vi "Enviar_configEstacion_Arduino.vi"(0 "VISA resource name":refnum<visa-resource-name>, 5 "Configuracion Estación":T1={"Coordenadas_estacion"={"Coord.Bandeja entrada"={"Coord. X0 entrada"=0, "Coord. Y0 entrada "=0, "Altura Z entrada"=0}, "Coord.Bandeja OK"={"Coord. X0 OK"=0, "Coord. Y0 OK"=0, "Altura Z OK"=0}, "Coord.Bandeja entrada FAIL"={"Coord. X0 FAIL"=0, "Coord. Y0 FAIL"=0, "Altura Z FAIL"=0}, "Coord. Socket"={"Coord. X socket"=0, "Coord. Y socket"=0, "Altura Z socket"=0}}, "Nombre Bandeja"="", "Datos bandeja"={"Nº de columnas "=0, "Nº de filas "=0, "largo"=0, "ancho"=0, "nombre"="nombre", "Paso X (en mm)"=0.0, "Paso Y (en mm)"=0.0, "DISTANCIA SUELO A CHIP  "=0.0, "Nº de celdas totales"=0, "Distancia chips bandejas contiguas"=0.0}}, 11 "error in (no error)":errorcluster) -> (4 "trama datos enviada":string, 6 "datos enviados = datos leídos?":bool, 10 "datos leídos":string, 15 "error IO":errorcluster)   [LabVIEW 2019]
uses:
  LVPROJ_CONFIG_ESTACION/Type_defs/Coordenadas_estacion.ctl
  LVPROJ_CREAR BANDEJAS/Type_defs/Data_Bandeja.ctl
  <vilib>/Utility/error.llb/Error Cluster From Error Code.vi
  <vilib>/ErrorRing/Error Ring.xnode
  SHARED VI'S/SHARED VI'S.lvlib
panel:
  out "return count":u32
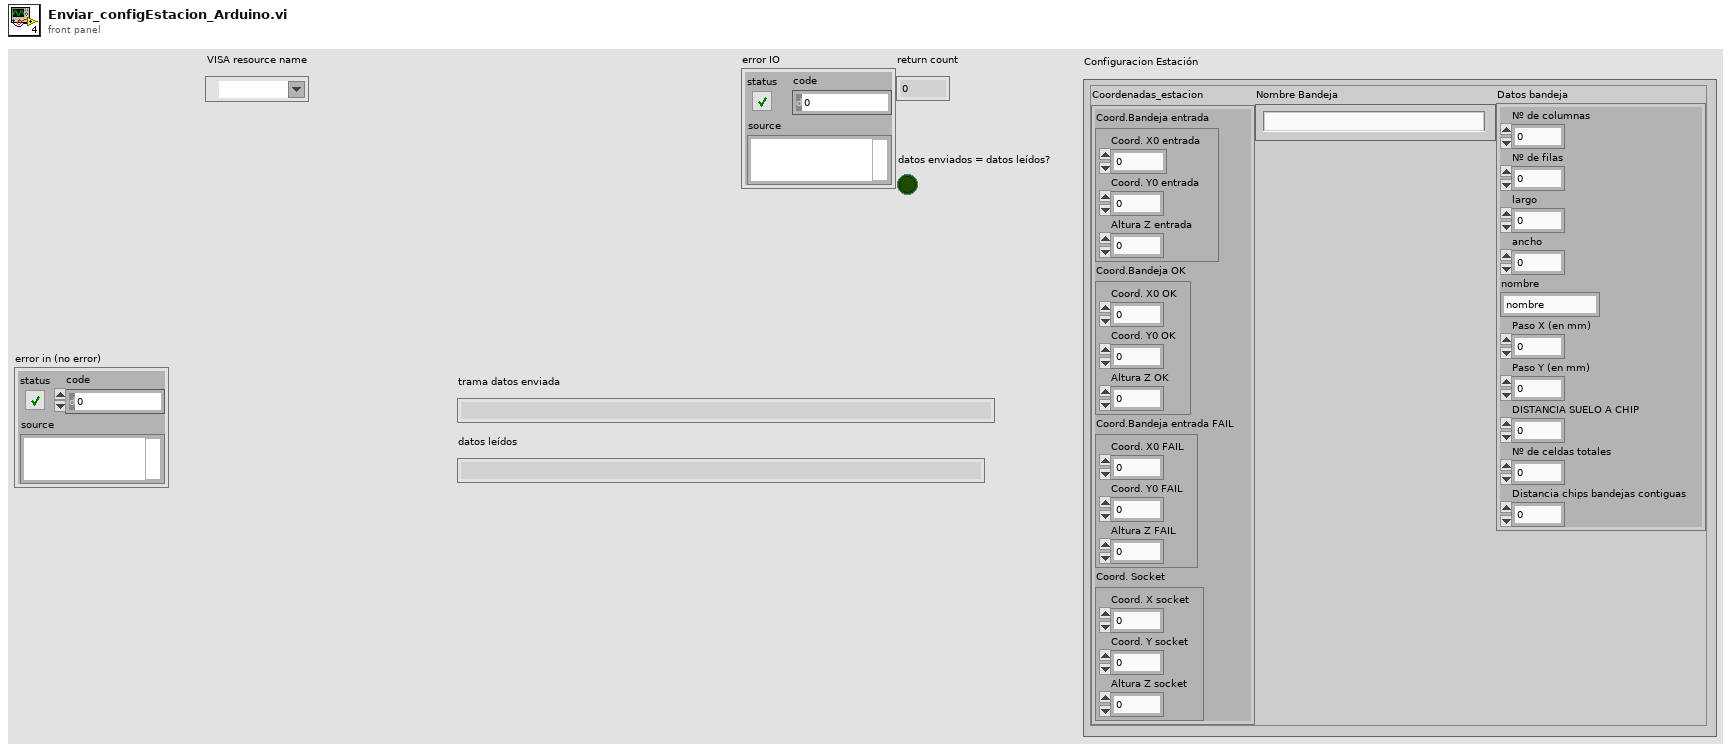
[diagram p1: front panel]
types:
  T1 = typedef "Configuracion_estación.ctl" = cluster{"Coordenadas_estacion":T2, "Nombre Bandeja":string, "Datos bandeja":T3}
  T2 = typedef "Coordenadas_estacion.ctl" = cluster{"Coord.Bandeja entrada":cluster{"Coord. X0 entrada":u32, "Coord. Y0 entrada ":u32, "Altura Z entrada":u32}, "Coord.Bandeja OK":cluster{"Coord. X0 OK":u32, "Coord. Y0 OK":u32, "Altura Z OK":u32}, "Coord.Bandeja entrada FAIL":cluster{"Coord. X0 FAIL":u32, "Coord. Y0 FAIL":u32, "Altura Z FAIL":u32}, "Coord. Socket":cluster{"Coord. X socket":u32, "Coord. Y socket":u32, "Altura Z socket":u32}}
  T3 = typedef "Data_Bandeja.ctl" = cluster{"Nº de columnas ":u32, "Nº de filas ":u32, "largo":u32, "ancho":u32, "nombre":string, "Paso X (en mm)":dbl, "Paso Y (en mm)":dbl, "DISTANCIA SUELO A CHIP  ":dbl, "Nº de celdas totales":u16, "Distancia chips bandejas contiguas":dbl}
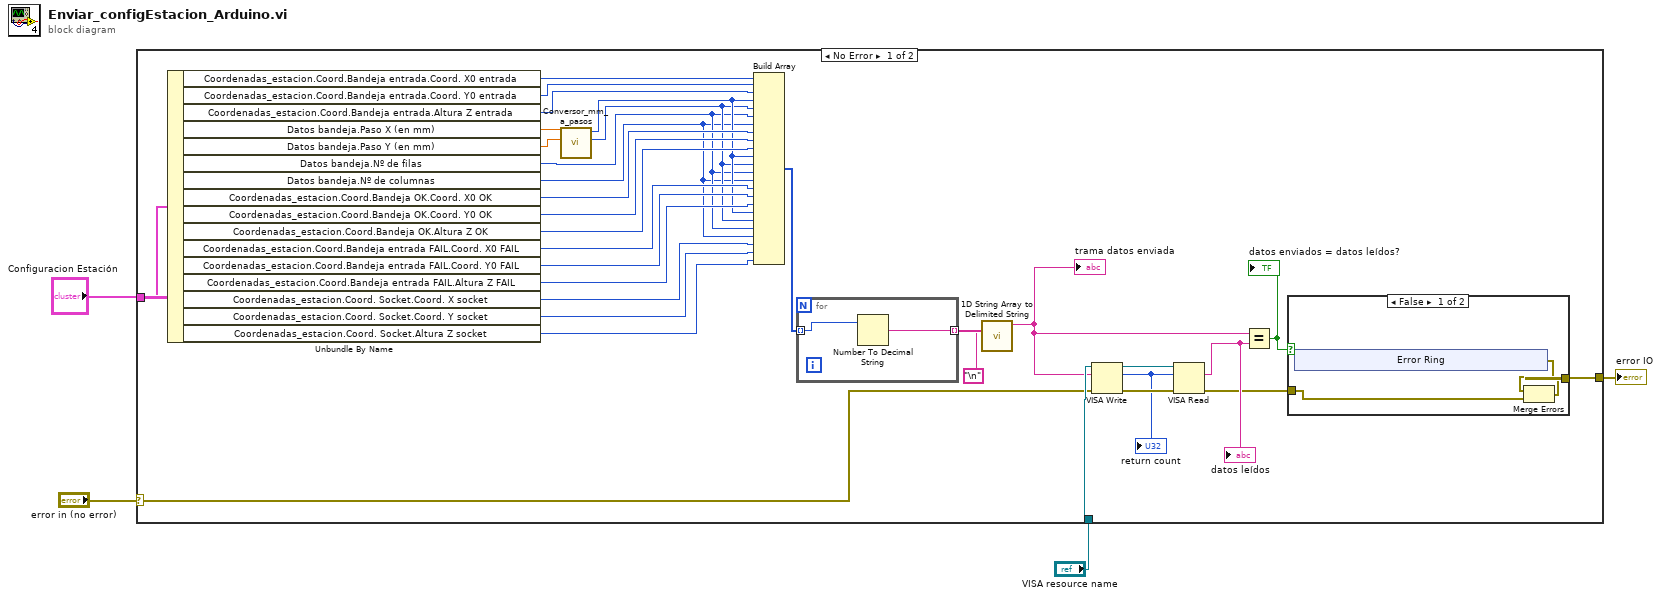
[diagram p0: block diagram]
diagram:
  n1 = case shown="No Error" "error in (no error)" {
    selector: "error in (no error)" -> [w30 w48]
    tunnel: "Configuracion Estación" -> [w36 _]
    tunnel: "VISA resource name" -> [w31 _]
    tunnel: [w23 w48] -> w1
    frame No Error {
      n2 = Unbundle By Name(w36) -> ("Coordenadas_estacion.Coord.Bandeja entrada.Coord. X0 entrada"=w35:u32, "Coordenadas_estacion.Coord.Bandeja entrada.Coord. Y0 entrada"=w21:u32, "Coordenadas_estacion.Coord.Bandeja entrada.Altura Z entrada"=w20:u32, "Datos bandeja.Paso X (en mm)"=w19:dbl, "Datos bandeja.Paso Y (en mm)"=w18:dbl, "Datos bandeja.Nº de filas"=w9:u32, "Datos bandeja.Nº de columnas"=w8:u32, "Coordenadas_estacion.Coord.Bandeja OK.Coord. X0 OK"=w17:u32, "Coordenadas_estacion.Coord.Bandeja OK.Coord. Y0 OK"=w16:u32, "Coordenadas_estacion.Coord.Bandeja OK.Altura Z OK"=w15:u32, "Coordenadas_estacion.Coord.Bandeja entrada FAIL.Coord. X0 FAIL"=w14:u32, "Coordenadas_estacion.Coord.Bandeja entrada FAIL.Coord. Y0 FAIL"=w13:u32, "Coordenadas_estacion.Coord.Bandeja entrada FAIL.Altura Z FAIL"=w12:u32, "Coordenadas_estacion.Coord. Socket.Coord. X socket"=w7:u32, "Coordenadas_estacion.Coord. Socket.Coord. Y socket"=w6:u32, "Coordenadas_estacion.Coord. Socket.Altura Z socket"=w5:u32)
      n3 = call "Conversor_mm_a_pasos.vi"("pasosY"=w18, "pasosX"=w19) -> ("PASOS EN Y"=w10:u32, "PASOS EN X"=w11:u32)  [unwired: 6 in, 2 out]
      n4 = Build Array(w35, w21, w20, w11, w10, w9, w8, w17, w16, w15, w11, w10, w9, w8, w14, w13, w12, w11, w10, w9, w8, w7, w6, w5) -> (w34:u32[])
      n5 = for {
        tunnel: w34 -> [w47] mode=indexing
        tunnel: [w46] -> w33 mode=indexing
        n6 = Number To Decimal String(number=w47) -> (decimal integer string=w46:string)  [unwired: 1 in]
      }
      n7 = call <vilib>:"1D String Array to Delimited String.vi"("delimiter"="\n", "string array"=w33) -> ("delimited string"=w26:string)  [unwired: 9 in]
      "trama datos enviada" <- w26
      n8 = VISA Write(VISA resource name=w31, write buffer=w26, error in (no error)=w30) -> (VISA resource name out=w28:refnum<visa-resource-name>, return count=w27:u32, error out=w29:errorcluster)
      "return count" <- w27
      n9 = VISA Read(VISA resource name=w28, byte count=w27, error in (no error)=w29) -> (read buffer=w25:string, error out=w22:errorcluster)  [unwired: 2 out]
      "datos leídos" <- w25
      n10 = Equal?(x=w26, y=w25) -> (x = y?=w24:bool)
      "datos enviados = datos leídos?" <- w24
      n11 = case shown="False" w24 {
        tunnel: [w39 w45] -> w23
        tunnel: w22 -> [w37 w45]
        frame False {
          n12 = xnode "Error Ring"() -> ("error out"=w38:errorcluster)
          n13 = Merge Errors(w38, w37) -> (w39:errorcluster)
        }
        frame True {
        }
      }
    }
    frame Error {
    }
  }
  "error IO" <- w1
